vi "NewCore.vi"(8 "error in (no error)":errorcluster, 10 "ParamsArray":variant[](array[variant]), 11 "ConcreteProductA in":refnum<class "ConcreteProductA.lvclass">) -> (0 "error out":errorcluster, 3 "ConcreteProductA out":refnum<class "ConcreteProductA.lvclass">)   [LabVIEW 2020, in "FactoryMethod.lvlib" / "ConcreteProductA.lvclass"]
uses:
  ConcreteProductA.lvclass
  Private/TypeDef/privateData.ctl
  ConcreteProductA.lvclass/ConcreteProductA.ctl
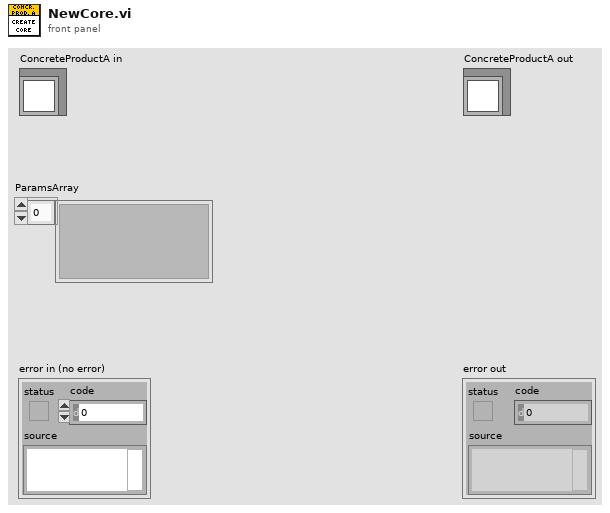
[diagram p1: front panel]
types:
  T1 = typedef "FactoryMethod.lvlib/ConcreteProductA.lvclass/privateData.ctl" = cluster{"Dummy":i32}
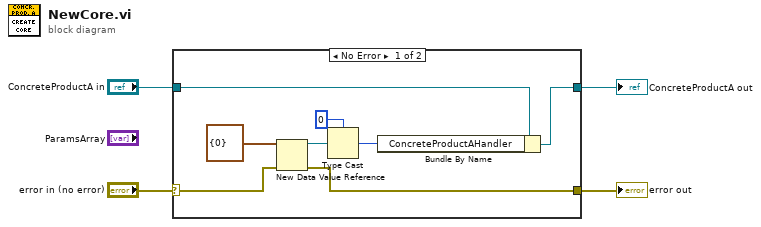
[diagram p0: block diagram]
diagram:
  n1 = case shown="No Error" "error in (no error)" {
    selector: "error in (no error)" -> [w6 w14]
    tunnel: [w7 w14] -> w1
    tunnel: [w9 w13] -> w3
    tunnel: "ConcreteProductA in" -> [w8 w13]
    frame No Error {
      n2 = New Data Value Reference(data value=T1 {"Dummy"=0} ("privateData"), error in=w6) -> (data value reference=w12:refnum<data-value>, error out=w7:errorcluster)
      n3 = Type Cast(type=u32 0, x=w12) -> (*(type *) &x=w10:u32)
      n4 = Bundle By Name(cluster=w8, "ConcreteProductAHandler"=w10) -> (w9:refnum<class "ConcreteProductA.lvclass">)
    }
    frame Error {
    }
  }
  "error out" <- w1
  "ConcreteProductA out" <- w3
